vi "DetectAndConnectLasers.vi"(8 "error in (no error)":errorcluster, 11 "Config In":T1 {"Hardware Configuration"."Lasers Configuration"."SettingValues"."785 Power" format="%.1f"; "Hardware Configuration"."Lasers Configuration"."SettingValues"."647 Power" format="%.1f"; "Hardware Configuration"."Lasers Configuration"."SettingValues"."561 Power" format="%.1f"; "Hardware Configuration"."Lasers Configuration"."SettingValues"."532 Power" format="%.1f"; "Hardware Configuration"."Lasers Configuration"."SettingValues"."488 Power" format="%.1f"; "Hardware Configuration"."Lasers Configuration"."SettingValues"."405 Power" format="%.1f"}) -> (0 "error out":errorcluster, 3 "Config Out":T1 {"Hardware Configuration"."Lasers Configuration"."SettingValues"."785 Power" format="%.1f"; "Hardware Configuration"."Lasers Configuration"."SettingValues"."647 Power" format="%.1f"; "Hardware Configuration"."Lasers Configuration"."SettingValues"."561 Power" format="%.1f"; "Hardware Configuration"."Lasers Configuration"."SettingValues"."532 Power" format="%.1f"; "Hardware Configuration"."Lasers Configuration"."SettingValues"."488 Power" format="%.1f"; "Hardware Configuration"."Lasers Configuration"."SettingValues"."405 Power" format="%.1f"})   [LabVIEW 2019]
uses:
  Settings/Settings.ctl
  Support/Hardware Configuration.ctl
  Support/Camera Configuration.ctl
  D:/SDK/PMQI-LabViewSamples/Examples/Dependencies/PVCamNET.dll
  <vilib>/userdefined/High Color/IMAQdx.ctl
  E:/DevHardSoftware/MMicroscopy/HardwareAdapter/Lasers/Dependencies/Oxxius_Boxx.dll
  Dependencies/Oxxius_Boxx.dll
  Logging/Logging Configuration.ctl
  controls/UI Configuration.ctl
  controls/CallBack Refs.ctl
  Logging/Logging.lvlib
  Settings/Settings.lvlib
panel:
  out "Name":string
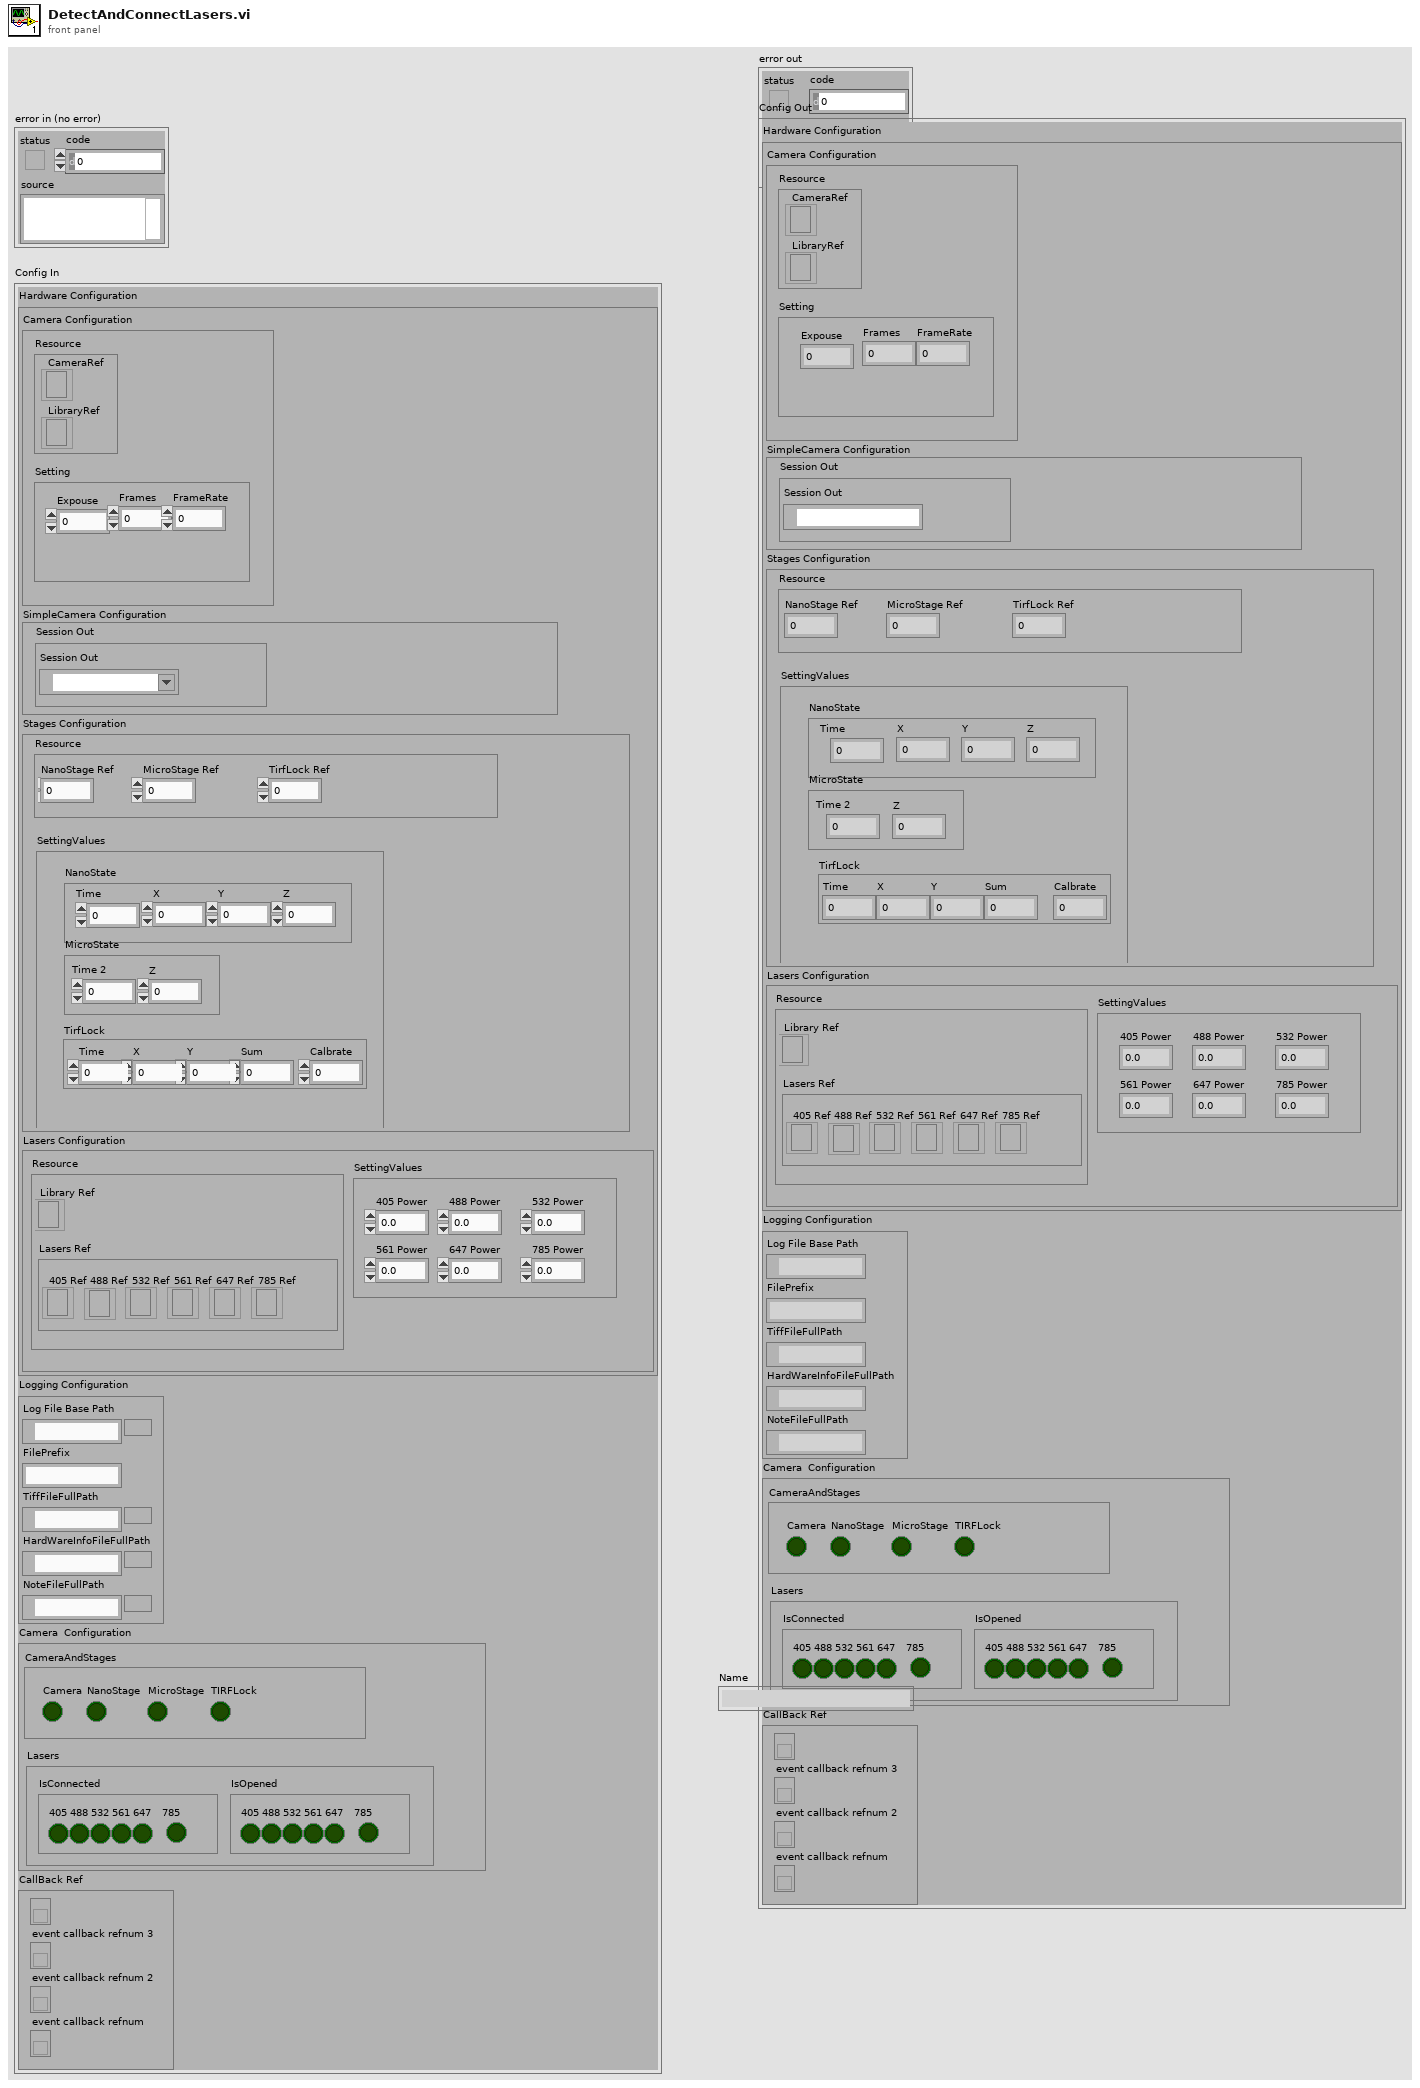
[diagram p1: front panel]
types:
  T1 = typedef "Settings.lvlib/Settings.ctl" = cluster{"Hardware Configuration":T2, "Logging Configuration":T5, "HardWare Status":cluster{"CameraAndStages":T6, "Lasers":cluster{"IsConnected":cluster{"405":bool, "488":bool, "532":bool, "561":bool, "647":bool, "785":bool}, "IsOpened":cluster{"405":bool, "488":bool, "532":bool, "561":bool, "647":bool, "785":bool}}}, "CallBack Ref":T7}
  T2 = typedef "Hardware Configuration.ctl" = cluster{"Camera Configuration":T3, "SimpleCamera Configuration":cluster{"Resource":cluster{"Session Out":T4}}, "Stages Configuration":cluster{"Resource":cluster{"NanoStage Ref":i32, "MicroStage Ref":i32, "TirfLock Ref":i32}, "SettingValues":cluster{"NanoState":cluster{"Time":dbl, "X":dbl, "Y":dbl, "Z":dbl}, "MicroState":cluster{"Time 2":dbl, "Z":dbl}, "TirfLock":cluster{"Time":dbl, "X":dbl, "Y":dbl, "Sum":dbl, "Calbrate":dbl}}}, "Lasers Configuration":cluster{"SettingValues":cluster{"405 Power":sgl, "488 Power":sgl, "532 Power":sgl, "561 Power":sgl, "647 Power":sgl, "785 Power":sgl}, "Resource":cluster{"Library Ref":refnum<k24>, "Lasers Ref":cluster{"405 Ref":refnum<k24>, "488 Ref":refnum<k24>, "532 Ref":refnum<k24>, "561 Ref":refnum<k24>, "647 Ref":refnum<k24>, "785 Ref":refnum<k24>}}}}
  T3 = typedef "Camera Configuration.ctl" = cluster{"Resource":cluster{"CameraRef":refnum<k24>, "LibraryRef":refnum<k24>}, "Setting":cluster{"Expouse":dbl, "Frames":dbl, "FrameRate":dbl}}
  T4 = typedef "IMAQdx.ctl" = refnum<k21>
  T5 = typedef "Logging.lvlib/Logging Configuration.ctl" = cluster{"Log File Base Path":path, "FilePrefix":string, "TiffFileFullPath":path, "HardWareInfoFileFullPath":path, "NoteFileFullPath":path}
  T6 = typedef "UI Configuration.ctl" = cluster{"Camera":bool, "NanoStage":bool, "MicroStage":bool, "TIRFLock":bool}
  T7 = typedef "CallBack Refs.ctl" = cluster{"event callback refnum":refnum<k27>, "event callback refnum 2":refnum<k27>, "event callback refnum 3":refnum<k27>, "event callback refnum 4":refnum<k27>}
  T8 = cluster{"405":bool, "488":bool, "532":bool, "561":bool, "647":bool, "785":bool}
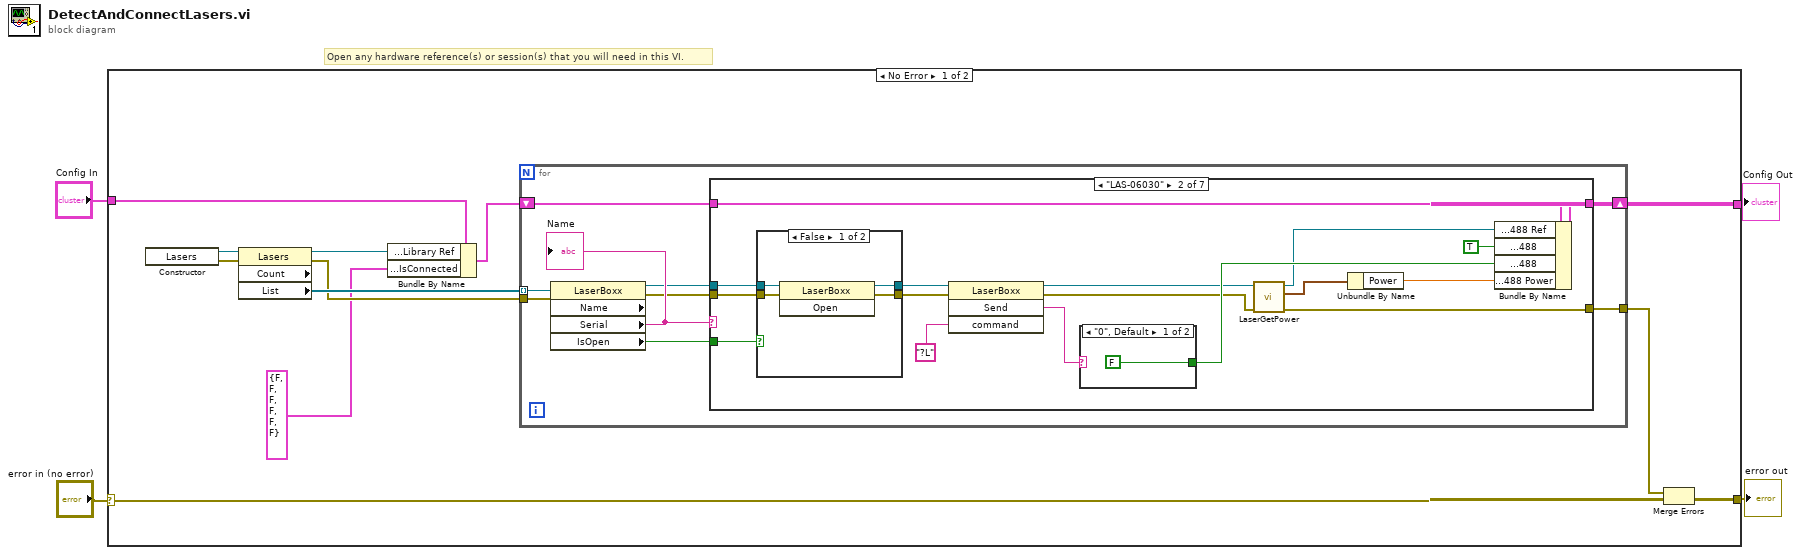
[diagram p0: block diagram]
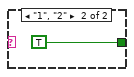
[diagram p3: hidden frame]
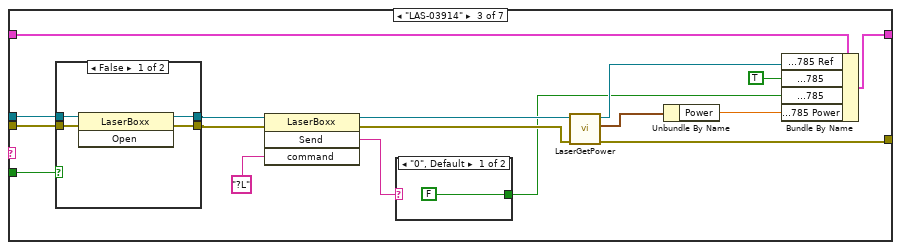
[diagram p5: hidden frame]
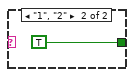
[diagram p6: hidden frame]
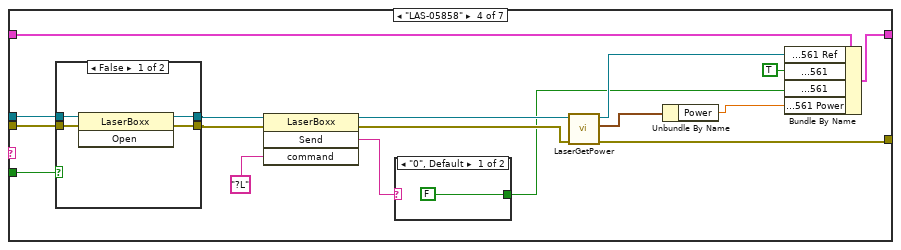
[diagram p8: hidden frame]
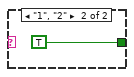
[diagram p9: hidden frame]
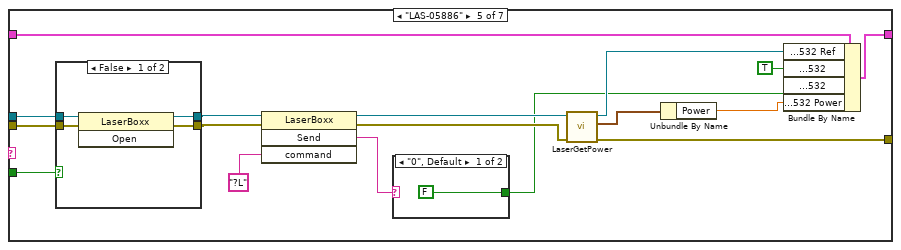
[diagram p11: hidden frame]
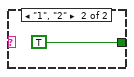
[diagram p12: hidden frame]
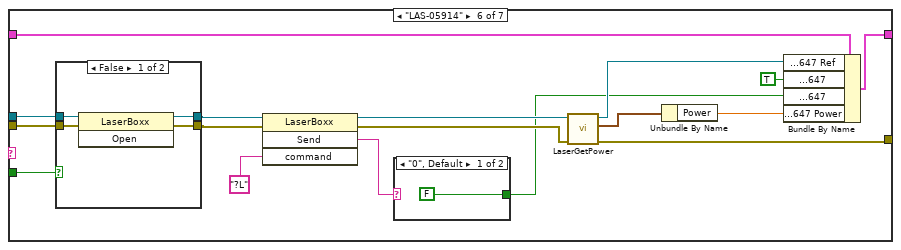
[diagram p14: hidden frame]
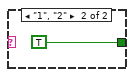
[diagram p15: hidden frame]
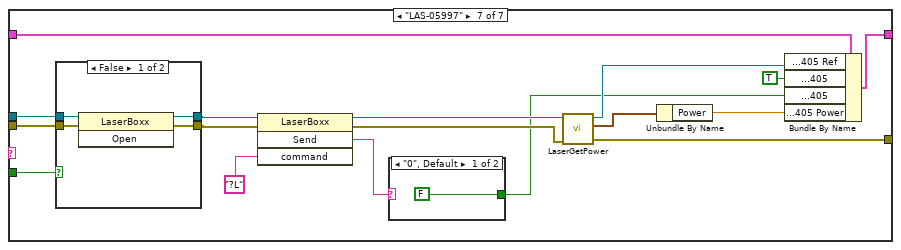
[diagram p17: hidden frame]
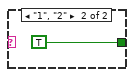
[diagram p18: hidden frame]
diagram:
  # "Open any hardware reference(s) or session(s) that you will need in this VI."
  n1 = case shown="No Error" "error in (no error)" {
    selector: "error in (no error)" -> [w15 w178]
    tunnel: [w16 w178] -> w1
    tunnel: "Config In" -> [w8 w179]
    tunnel: [w5 w179] -> w2
    frame No Error {
      n2 = constructor class="Lasers"() -> (reference out=w13:refnum<k24>, error out=w12:errorcluster)  [unwired: 3 in, 1 out]
      n3 = property class="Lasers" props=["Count", "List"](reference=w13, error in=w12) -> (reference out=w10:refnum<k24>, error out=w11:errorcluster, "List"=w14:refnum<k24>[])  [unwired: 1 out]
      n4 = Bundle By Name(cluster=w8, "Hardware Configuration.Lasers Configuration.Resource.Library Ref"=w10, "HardWare Status.Lasers.IsConnected"=T8 {"405"=FALSE, "488"=FALSE, "532"=FALSE, "561"=FALSE, "647"=FALSE, "785"=FALSE}) -> (w7:T1)
      n5 = for {
        tunnel: w14 -> [w25] mode=indexing
        tunnel: w11 -> [w24]
        tunnel: [w23] -> w9
        shift-right: [w17] -> w5
        shift-left: w7 -> [w18]
        n6 = property class="LaserBoxx" props=["Name", "Serial", "IsOpen"](reference=w25, error in=w24) -> (reference out=w21:refnum<k24>, error out=w20:errorcluster, "Serial"=w22:string, "IsOpen"=w19:bool)  [unwired: 1 out]
        "Name" <- w22
        n7 = case shown="\"LAS-06030\"" w22 {
          tunnel: w20 -> [w27 w44 w69 w94 w119 w144 w169]
          tunnel: [w27 w31 w53 w78 w106 w128 w153] -> w23
          tunnel: w21 -> [_ w40 w65 w90 w115 w140 w165]
          tunnel: w19 -> [_ w43 w68 w93 w118 w143 w168]
          tunnel: w18 -> [w26 w42 w67 w92 w117 w142 w167]
          tunnel: [w26 w41 w66 w91 w116 w141 w166] -> w17
          frame Default {
          }
          frame "LAS-06030" {
            n8 = case shown="False" w43 {
              tunnel: w44 -> [w50 w52]
              tunnel: w40 -> [w49 w51]
              tunnel: [w48 w52] -> w37
              tunnel: [w47 w51] -> w36
              frame False {
                n9 = invoke class="LaserBoxx" method="Open"(reference=w49, error in=w50) -> (reference out=w47:refnum<k24>, error out=w48:errorcluster)  [unwired: 1 in, 1 out]
              }
              frame True {
              }
            }
            n10 = invoke class="LaserBoxx" method="Send"(reference=w36, error in=w37, "command"="?L") -> (reference out=w32:refnum<k24>, error out=w33:errorcluster, "Send"=w35:string)  [unwired: 1 in, 1 out]
            n11 = case shown="\"0\", Default" w35 {
              tunnel: [FALSE TRUE] -> w34
              frame "0", Default {
              }
              frame "1", "2" {
              }
            }
            n12 = call "LaserGetPower.vi"("error in (no error)"=w33, "reference In"=w32) -> ("error out"=w31:errorcluster, "Power"=w29:cluster{"Time":dbl, "Power":dbl}, "reference out"=w30:refnum<k24>)  [unwired: 6 in]
            n13 = Unbundle By Name(w29) -> ("Power"=w28:dbl)
            n14 = Bundle By Name(cluster=w42, "Hardware Configuration.Lasers Configuration.Resource.Lasers Ref.488 Ref"=w30, "HardWare Status.Lasers.IsConnected.488"=TRUE ("HardWare Status.Lasers.IsConnected.405"), "HardWare Status.Lasers.IsOpened.488"=w34, "Hardware Configuration.Lasers Configuration.SettingValues.488 Power"=w28) -> (w41:T1)
          }
          frame "LAS-03914" {
            n15 = case shown="False" w68 {
              tunnel: w69 -> [w75 w77]
              tunnel: w65 -> [w74 w76]
              tunnel: [w73 w77] -> w57
              tunnel: [w72 w76] -> w58
              frame False {
                n16 = invoke class="LaserBoxx" method="Open"(reference=w74, error in=w75) -> (reference out=w72:refnum<k24>, error out=w73:errorcluster)  [unwired: 1 in, 1 out]
              }
              frame True {
              }
            }
            n17 = invoke class="LaserBoxx" method="Send"(reference=w58, error in=w57, "command"="?L") -> (reference out=w60:refnum<k24>, error out=w61:errorcluster, "Send"=w62:string)  [unwired: 1 in, 1 out]
            n18 = case shown="\"0\", Default" w62 {
              tunnel: [FALSE TRUE] -> w55
              frame "0", Default {
              }
              frame "1", "2" {
              }
            }
            n19 = call "LaserGetPower.vi"("error in (no error)"=w61, "reference In"=w60) -> ("error out"=w53:errorcluster, "Power"=w59:cluster{"Time":dbl, "Power":dbl}, "reference out"=w56:refnum<k24>)  [unwired: 6 in]
            n20 = Unbundle By Name(w59) -> ("Power"=w54:dbl)
            n21 = Bundle By Name(cluster=w67, "Hardware Configuration.Lasers Configuration.Resource.Lasers Ref.785 Ref"=w56, "HardWare Status.Lasers.IsConnected.785"=TRUE ("HardWare Status.Lasers.IsConnected.405"), "HardWare Status.Lasers.IsOpened.785"=w55, "Hardware Configuration.Lasers Configuration.SettingValues.785 Power"=w54) -> (w66:T1)
          }
          frame "LAS-05858" {
            n22 = case shown="False" w93 {
              tunnel: w94 -> [w100 w102]
              tunnel: w90 -> [w99 w101]
              tunnel: [w98 w102] -> w82
              tunnel: [w97 w101] -> w83
              frame False {
                n23 = invoke class="LaserBoxx" method="Open"(reference=w99, error in=w100) -> (reference out=w97:refnum<k24>, error out=w98:errorcluster)  [unwired: 1 in, 1 out]
              }
              frame True {
              }
            }
            n24 = invoke class="LaserBoxx" method="Send"(reference=w83, error in=w82, "command"="?L") -> (reference out=w85:refnum<k24>, error out=w86:errorcluster, "Send"=w87:string)  [unwired: 1 in, 1 out]
            n25 = case shown="\"0\", Default" w87 {
              tunnel: [FALSE TRUE] -> w80
              frame "0", Default {
              }
              frame "1", "2" {
              }
            }
            n26 = call "LaserGetPower.vi"("error in (no error)"=w86, "reference In"=w85) -> ("error out"=w78:errorcluster, "Power"=w84:cluster{"Time":dbl, "Power":dbl}, "reference out"=w81:refnum<k24>)  [unwired: 6 in]
            n27 = Unbundle By Name(w84) -> ("Power"=w79:dbl)
            n28 = Bundle By Name(cluster=w92, "Hardware Configuration.Lasers Configuration.Resource.Lasers Ref.561 Ref"=w81, "HardWare Status.Lasers.IsConnected.561"=TRUE ("HardWare Status.Lasers.IsConnected.405"), "HardWare Status.Lasers.IsOpened.561"=w80, "Hardware Configuration.Lasers Configuration.SettingValues.561 Power"=w79) -> (w91:T1)
          }
          frame "LAS-05886" {
            n29 = case shown="False" w118 {
              tunnel: w119 -> [w125 w127]
              tunnel: w115 -> [w124 w126]
              tunnel: [w123 w127] -> w107
              tunnel: [w122 w126] -> w108
              frame False {
                n30 = invoke class="LaserBoxx" method="Open"(reference=w124, error in=w125) -> (reference out=w122:refnum<k24>, error out=w123:errorcluster)  [unwired: 1 in, 1 out]
              }
              frame True {
              }
            }
            n31 = invoke class="LaserBoxx" method="Send"(reference=w108, error in=w107, "command"="?L") -> (reference out=w110:refnum<k24>, error out=w111:errorcluster, "Send"=w112:string)  [unwired: 1 in, 1 out]
            n32 = case shown="\"0\", Default" w112 {
              tunnel: [FALSE TRUE] -> w104
              frame "0", Default {
              }
              frame "1", "2" {
              }
            }
            n33 = call "LaserGetPower.vi"("error in (no error)"=w111, "reference In"=w110) -> ("error out"=w106:errorcluster, "Power"=w109:cluster{"Time":dbl, "Power":dbl}, "reference out"=w105:refnum<k24>)  [unwired: 6 in]
            n34 = Unbundle By Name(w109) -> ("Power"=w103:dbl)
            n35 = Bundle By Name(cluster=w117, "Hardware Configuration.Lasers Configuration.Resource.Lasers Ref.532 Ref"=w105, "HardWare Status.Lasers.IsConnected.532"=TRUE ("HardWare Status.Lasers.IsConnected.405"), "HardWare Status.Lasers.IsOpened.532"=w104, "Hardware Configuration.Lasers Configuration.SettingValues.532 Power"=w103) -> (w116:T1)
          }
          frame "LAS-05914" {
            n36 = case shown="False" w143 {
              tunnel: w144 -> [w150 w152]
              tunnel: w140 -> [w149 w151]
              tunnel: [w148 w152] -> w132
              tunnel: [w147 w151] -> w133
              frame False {
                n37 = invoke class="LaserBoxx" method="Open"(reference=w149, error in=w150) -> (reference out=w147:refnum<k24>, error out=w148:errorcluster)  [unwired: 1 in, 1 out]
              }
              frame True {
              }
            }
            n38 = invoke class="LaserBoxx" method="Send"(reference=w133, error in=w132, "command"="?L") -> (reference out=w135:refnum<k24>, error out=w136:errorcluster, "Send"=w137:string)  [unwired: 1 in, 1 out]
            n39 = case shown="\"0\", Default" w137 {
              tunnel: [FALSE TRUE] -> w130
              frame "0", Default {
              }
              frame "1", "2" {
              }
            }
            n40 = call "LaserGetPower.vi"("error in (no error)"=w136, "reference In"=w135) -> ("error out"=w128:errorcluster, "Power"=w134:cluster{"Time":dbl, "Power":dbl}, "reference out"=w131:refnum<k24>)  [unwired: 6 in]
            n41 = Unbundle By Name(w134) -> ("Power"=w129:dbl)
            n42 = Bundle By Name(cluster=w142, "Hardware Configuration.Lasers Configuration.Resource.Lasers Ref.647 Ref"=w131, "HardWare Status.Lasers.IsConnected.647"=TRUE ("HardWare Status.Lasers.IsConnected.405"), "HardWare Status.Lasers.IsOpened.647"=w130, "Hardware Configuration.Lasers Configuration.SettingValues.647 Power"=w129) -> (w141:T1)
          }
          frame "LAS-05997" {
            n43 = case shown="False" w168 {
              tunnel: w169 -> [w175 w177]
              tunnel: w165 -> [w174 w176]
              tunnel: [w173 w177] -> w157
              tunnel: [w172 w176] -> w158
              frame False {
                n44 = invoke class="LaserBoxx" method="Open"(reference=w174, error in=w175) -> (reference out=w172:refnum<k24>, error out=w173:errorcluster)  [unwired: 1 in, 1 out]
              }
              frame True {
              }
            }
            n45 = invoke class="LaserBoxx" method="Send"(reference=w158, error in=w157, "command"="?L") -> (reference out=w160:refnum<k24>, error out=w161:errorcluster, "Send"=w162:string)  [unwired: 1 in, 1 out]
            n46 = case shown="\"0\", Default" w162 {
              tunnel: [FALSE TRUE] -> w155
              frame "0", Default {
              }
              frame "1", "2" {
              }
            }
            n47 = call "LaserGetPower.vi"("error in (no error)"=w161, "reference In"=w160) -> ("error out"=w153:errorcluster, "Power"=w159:cluster{"Time":dbl, "Power":dbl}, "reference out"=w156:refnum<k24>)  [unwired: 6 in]
            n48 = Unbundle By Name(w159) -> ("Power"=w154:dbl)
            n49 = Bundle By Name(cluster=w167, "Hardware Configuration.Lasers Configuration.Resource.Lasers Ref.405 Ref"=w156, "HardWare Status.Lasers.IsConnected.405"=TRUE, "HardWare Status.Lasers.IsOpened.405"=w155, "Hardware Configuration.Lasers Configuration.SettingValues.405 Power"=w154) -> (w166:T1)
          }
        }
      }
      n50 = Merge Errors(w9, w15) -> (w16:errorcluster)
    }
    frame Error {
    }
  }
  "error out" <- w1
  "Config Out" <- w2
